vi "Functional Test.vi"() -> ()   [LabVIEW 2023]
uses:
  <vilib>/Utility/file.llb/Read Delimited Spreadsheet (string).vi
panel:
  in  "Halt Run":bool=TRUE
  out "System Info":string[][](array[string])
  out "System":string
  in  "Exit":bool=TRUE
  in  "Start":bool=TRUE
  out "Frequency Address":i16=8
  in  "System Status":string
  out "Functional Test Data":string
  # "Aging System 1 Functional Test"
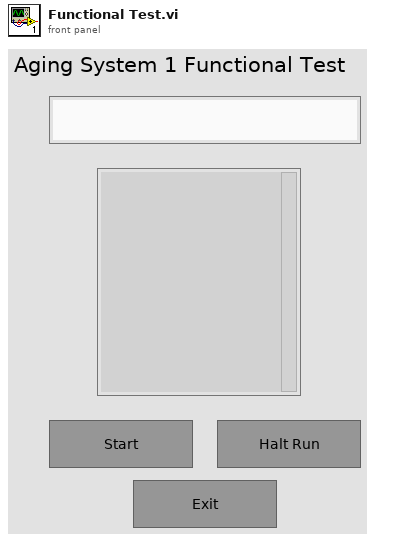
[diagram p1: front panel]
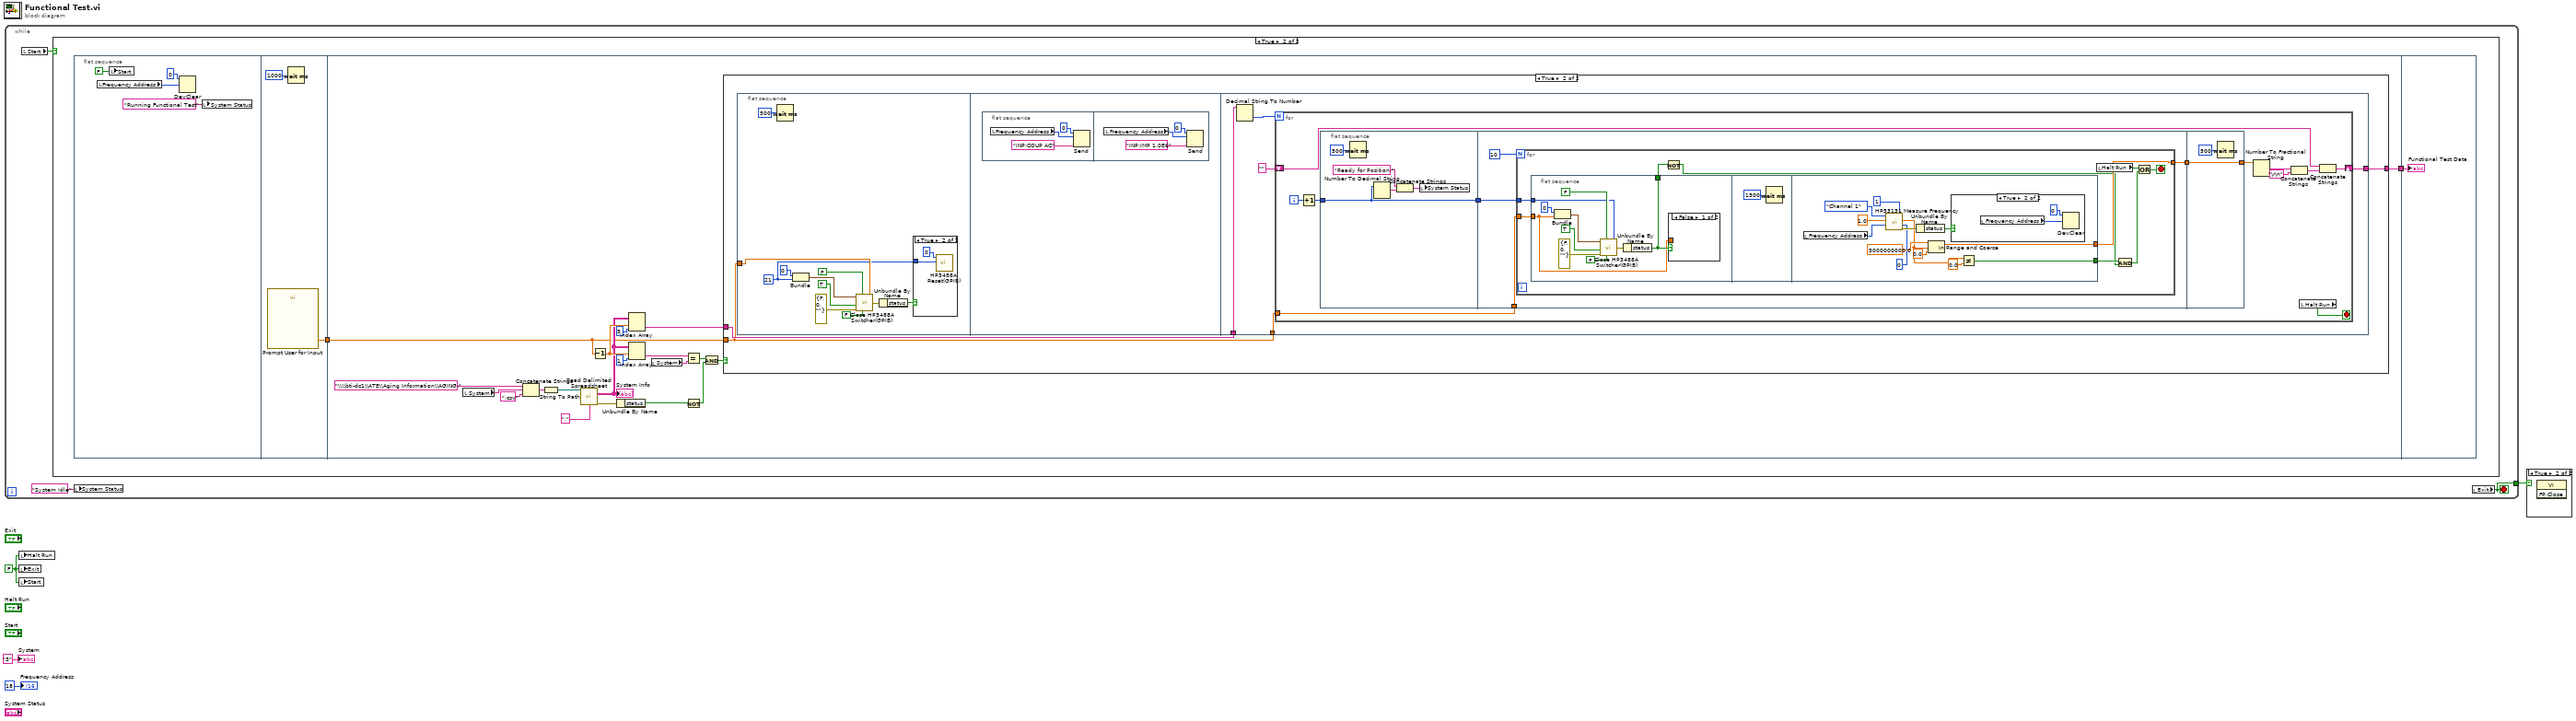
[diagram p0: block diagram]
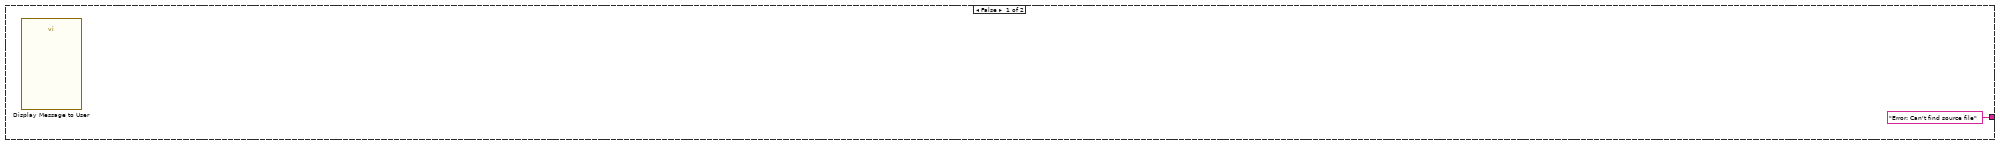
[diagram p4: hidden frame]
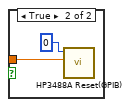
[diagram p6: hidden frame]
diagram:
  w3 = FALSE ("Exit")
  n1 = while {
    tunnel: [w6] -> w1
    stop <- w6 stop-if-true
    n2 = local read "Start"() -> (w7:bool)
    n3 = case shown="True" w7 {
      frame False {
      }
      frame True {
        n4 = flat-sequence {
          tunnel: [w14] -> w8
          tunnel: [w28] -> w9
          tunnel: w8 -> [w16]
          tunnel: w9 -> [w124]
          frame #0 {
            n5 = local read "Frequency Address"() -> (w12:i16)
            n6 = local write "Start"(FALSE ("Start")) -> ()
            n7 = DevClear(3:w12, 4:0 ("GPIB Bus")) -> ()  [unwired: 1 in, 2 out]
            n8 = local write "System Status"("Running Functional Test" ("System Status")) -> ()
          }
          frame #1 {
            n9 = call "Prompt User for Input"() -> ("Rack Number:"=w14:dbl)  [unwired: 17 in, 2 out]
            n10 = Wait (ms)(milliseconds to wait=u32 1000) -> ()  [unwired: 1 out]
          }
          frame #2 {
            n11 = local read "System"() -> (w33:string)
            n12 = Concatenate Strings("\\\\bti-dc1\\ATE\\Aging Information\\AGING-" ("string"), w33, ".csv" ("string")) -> (w32:string)
            n13 = String To Path(string=w32) -> (path=w21:path)
            n14 = call-poly <vilib>:"Read Delimited Spreadsheet.vi"("file path (dialog if empty)"=w21, "delimiter (\\t)"="," ("delimiter (\\t)")) -> ("all rows"=w20:string[][], "error out"=w19:errorcluster)  [unwired: 8 in, 4 out]
            "System Info" <- w20
            n15 = Decrement(x=w16) -> (x-1=w22:dbl)
            n16 = Unbundle By Name(w19) -> ("status"=w31:bool)
            n17 = Index Array(array=w20, index (row)=w22, index (col)=5 ("disabled index (col)")) -> (element=w29:string)
            n18 = Index Array(array=w20, index (row)=w22, index (col)=1 ("disabled index (col)")) -> (element=w26:string)
            n19 = local read "System"() -> (w17:string)
            n20 = Equal?(x=w26, y=w17) -> (x = y?=w25:bool)
            n21 = Not(x=w31) -> (.not. x?=w24:bool)
            n22 = And(x=w25, y=w24) -> (x .and. y?=w23:bool)
            n23 = case shown="True" w23 {
              tunnel: w29 -> [_ w38]
              tunnel: ["Error: Can't find source file" w39] -> w28
              tunnel: w16 -> [_ w37]
              frame False {
                n24 = call "Display Message to User"() -> ()  [unwired: 10 in, 2 out]
              }
              frame True {
                n25 = flat-sequence {
                  tunnel: w37 -> [w41]
                  tunnel: [w62] -> w39
                  tunnel: w38 -> [w61]
                  tunnel: w37 -> [w59]
                  frame #0 {
                    w40 = 21 ("GPIB Bus")
                    n26 = Wait (ms)(milliseconds to wait=u32 500) -> ()  [unwired: 1 out]
                    n27 = Bundle("GPIB Bus"=0, "GPIB Bus"=w40) -> (w48:cluster{"GPIB Bus":i32, "GPIB Bus":i32})  [unwired: 1 in]
                    n28 = call "Close HP3488A Switcher(GPIB).vi"("Device In"=w48, "reset"=FALSE, "Use Card# 5"=TRUE, "ID query"=FALSE, "error in (no error)"=errorcluster {"status"=FALSE, "code"=0, "source"=""}, "Position Number"=w41) -> ("error out"=w49:errorcluster)  [unwired: 2 in]
                    n29 = Unbundle By Name(w49) -> ("status"=w47:bool)
                    n30 = case shown="True" w47 {
                      tunnel: w40 -> [_ w51]
                      frame False {
                      }
                      frame True {
                        n31 = call "HP3488A Reset(GPIB).vi"("Address"=w51, "GPIB#"=0 ("GPIB Bus")) -> ()  [unwired: 3 in, 1 out]
                      }
                    }
                  }
                  frame #1 {
                    n32 = flat-sequence {
                      frame #0 {
                        n33 = local read "Frequency Address"() -> (w53:i16)
                        n34 = Send(0:0 ("bus"), 2:w53, 5:"INP:COUP AC" ("data string")) -> ()  [unwired: 2 in, 3 out]
                      }
                      frame #1 {
                        n35 = local read "Frequency Address"() -> (w58:i16)
                        n36 = Send(0:0 ("bus"), 2:w58, 5:"INP:IMP 1.0E6" ("data string")) -> ()  [unwired: 2 in, 3 out]
                      }
                    }
                  }
                  frame #2 {
                    n37 = Decimal String To Number(string=w61) -> (number=w60:i32)  [unwired: 2 in, 1 out]
                    n38 = for {
                      N: w60 -> [_]
                      shift-right: [w74] -> w62
                      shift-left: "" -> [w73]
                      tunnel: w59 -> [w64]
                      i -> [w68]
                      stop <- w65 stop-if-true
                      n39 = Increment(x=w68) -> (x+1=w67:i32)
                      n40 = flat-sequence {
                        tunnel: w67 -> [w79]
                        tunnel: [w79] -> w69
                        tunnel: [w83] -> w66
                        tunnel: w69 -> [w84]
                        tunnel: w64 -> [w81]
                        tunnel: [w123] -> w75
                        tunnel: w66 -> [w123]
                        frame #0 {
                          n41 = Wait (ms)(milliseconds to wait=u32 500) -> ()  [unwired: 1 out]
                          n42 = Number To Decimal String(number=w79) -> (decimal integer string=w77:string)  [unwired: 1 in]
                          n43 = Concatenate Strings("Ready for Position ", w77) -> (w78:string)
                          n44 = local write "System Status"(w78) -> ()
                        }
                        frame #1 {
                          n45 = for {
                            N: 10 -> [_]
                            tunnel: w84 -> [w93]
                            tunnel: [w92] -> w83
                            tunnel: w81 -> [w85]
                            stop <- w86 stop-if-true
                            n46 = flat-sequence {
                              tunnel: w93 -> [w96]
                              tunnel: [w95] -> w89
                              tunnel: w85 -> [w94]
                              tunnel: [w112] -> w92
                              tunnel: [w109] -> w91
                              frame #0 {
                                n47 = Bundle("GPIB Bus"=0, "Rack Number:"=w94) -> (w102:cluster{"GPIB Bus":i32, "Rack Number:":dbl})  [unwired: 1 in]
                                n48 = call "Close HP3488A Switcher(GPIB).vi"("Device In"=w102, "reset"=FALSE, "Use Card# 5"=TRUE, "ID query"=FALSE, "error in (no error)"=errorcluster {"status"=FALSE, "code"=0, "source"=""}, "Position Number"=w96) -> ("error out"=w103:errorcluster)  [unwired: 2 in]
                                n49 = Unbundle By Name(w103) -> ("status"=w95:bool)
                                n50 = case shown="False" w95 {
                                tunnel: w94 -> [_ w104]
                                frame False {
                                }
                                frame True {
                                n51 = call "HP3488A Reset(GPIB).vi"("Address"=w104, "GPIB#"=0 ("GPIB Bus")) -> ()  [unwired: 3 in, 1 out]
                                }
                                }
                              }
                              frame #1 {
                                n52 = Wait (ms)(milliseconds to wait=u32 1500) -> ()  [unwired: 1 out]
                              }
                              frame #2 {
                                n53 = local read "Frequency Address"() -> (w119:i16)
                                n54 = call "HP53131 Measure Frequency.vi"("GPIB Bus"=0, "Number of Readings"=1, "GPIB Address"=w119, "Gate Time"=1.0, "Channel(1,2,3)"=enum16{"Channel 1", "Channel 2", "Channel 3"}."Channel 1") -> ("error out"=w118:errorcluster, "Frequency"=w110:dbl)  [unwired: 1 in]
                                n55 = Unbundle By Name(w118) -> ("status"=w117:bool)
                                n56 = In Range and Coerce(upper limit=5000000000.0, x=w110, lower limit=0.0) -> (coerced(x)=w112:dbl)  [unwired: 1 out]
                                n57 = case shown="True" w117 {
                                frame False {
                                }
                                frame True {
                                n58 = local read "Frequency Address"() -> (w120:i16)
                                n59 = DevClear(3:w120, 4:0 ("GPIB Bus")) -> ()  [unwired: 1 in, 2 out]
                                }
                                }
                                n60 = Not Equal?(x=w110, y=0.0) -> (x != y?=w109:bool)
                              }
                            }
                            n61 = Not(x=w89) -> (.not. x?=w90:bool)
                            n62 = local read "Halt Run"() -> (w88:bool)
                            n63 = And(x=w91, y=w90) -> (x .and. y?=w87:bool)
                            n64 = Or(x=w88, y=w87) -> (x .or. y?=w86:bool)
                          }
                        }
                        frame #2 {
                          n65 = Wait (ms)(milliseconds to wait=u32 500) -> ()  [unwired: 1 out]
                        }
                      }
                      n66 = Number To Fractional String(number=w75) -> (F-format string=w72:string)  [unwired: 3 in]
                      n67 = Concatenate Strings(w72, "\r\n") -> (w70:string)
                      n68 = local read "Halt Run"() -> (w65:bool)
                      n69 = Concatenate Strings(w73, w70) -> (w74:string)
                    }
                  }
                }
              }
            }
          }
          frame #3 {
            "Functional Test Data" <- w124
          }
        }
      }
    }
    n70 = local write "System Status"("System Idle" ("System Status")) -> ()
    n71 = local read "Exit"() -> (w6:bool)
  }
  n72 = local write "Halt Run"(w3) -> ()
  n73 = local write "Exit"(w3) -> ()
  n74 = local write "Start"(w3) -> ()
  n75 = case shown="True" w1 {
    frame False {
    }
    frame True {
      n76 = invoke class="VI" method="FP.Close"() -> ()  [unwired: 3 in, 3 out]
    }
  }
  "Frequency Address" <- i16 18 ("Frequency Address")
  "System" <- "3" ("System")
